vi "Find Lowest F-Cost.vi"(6 "Closed List In":T1(array[cluster]), 8 "error in (no error)":errorcluster, 10 "Open List":T1(array[cluster])) -> (0 "error out":errorcluster, 1 "Square with Parent":T2, 2 "Square":cluster{"X":dbl, "Y":dbl}, 3 "Open List Out":T1(array[cluster]), 4 "Closed List Out":T1(array[cluster]))   [LabVIEW 2009]
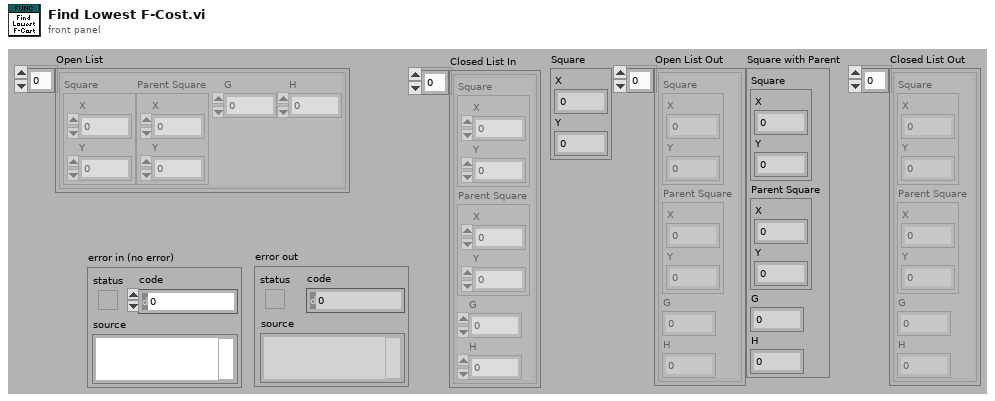
[diagram p1: front panel]
types:
  T1 = cluster{"Square":cluster{"X":dbl, "Y":dbl}, "Parent Square":cluster{"X":dbl, "Y":dbl}, "G":dbl, "H":dbl}[]
  T2 = cluster{"Square":cluster{"X":dbl, "Y":dbl}, "Parent Square":cluster{"X":dbl, "Y":dbl}, "G":dbl, "H":dbl}
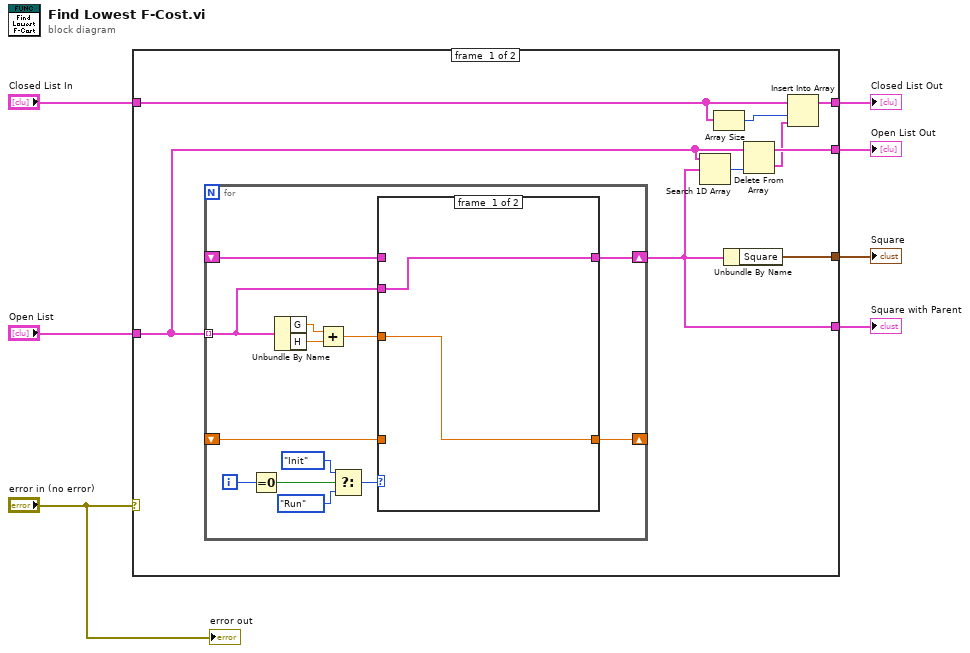
[diagram p0: block diagram]
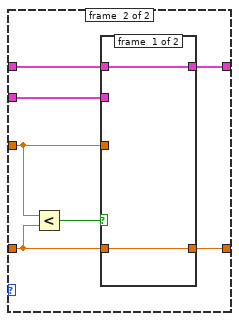
[diagram p2: hidden frame]
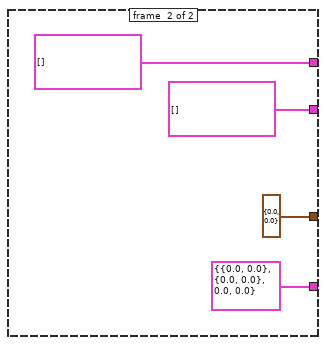
[diagram p4: hidden frame]
diagram:
  n1 = case shown="No Error" "error in (no error)" {
    tunnel: "Open List" -> [w16 _]
    tunnel: [w14 T1 [] ("Open List")] -> w5
    tunnel: [w13 cluster{"X":dbl, "Y":dbl} {"X"=0.0, "Y"=0.0} ("Square")] -> w4
    tunnel: [w12 T2 {"Square"={"X"=0.0, "Y"=0.0}, "Parent Square"={"X"=0.0, "Y"=0.0}, "G"=0.0, "H"=0.0} ("Cluster")] -> w3
    tunnel: "Closed List In" -> [w11 _]
    tunnel: [w8 T1 [] ("Closed List In")] -> w1
    frame #0 {
      n2 = for {
        tunnel: w16 -> [w19] mode=indexing
        shift-right: [w21] -> _
        shift-left: _ -> [w20]
        shift-right: [w18] -> w12
        shift-left: _ -> [w17]
        i -> [w24]
        n3 = Equal To 0?(x=w24) -> (x = 0?=w27:bool)
        n4 = Unbundle By Name(w19) -> ("G"=w29:dbl, "H"=w28:dbl)
        n5 = Add(x=w29, y=w28) -> (x+y=w22:dbl)
        n6 = Select(t=enum16{"Init", "Run"}."Init", s=w27, f=enum16{"Init", "Run"}."Run") -> (s? t:f=w23:enum16{"Init", "Run"})
        n7 = case shown="\"Run\"" w23 {
          tunnel: w22 -> [w31 w37]
          tunnel: [w31 w35] -> w21
          tunnel: w20 -> [_ w36]
          tunnel: w19 -> [w30 w32]
          tunnel: [w30 w34] -> w18
          tunnel: w17 -> [_ w33]
          frame #0 {
          }
          frame #1 {
            n8 = Less?(x=w37, y=w36) -> (x < y?=w38:bool)
            n9 = case shown="True" w38 {
              tunnel: w37 -> [_ w42]
              tunnel: w36 -> [w40 _]
              tunnel: [w40 w42] -> w35
              tunnel: [w39 w41] -> w34
              tunnel: w33 -> [w39 _]
              tunnel: w32 -> [_ w41]
              frame #0 {
              }
              frame #1 {
              }
            }
          }
        }
      }
      n10 = Search 1D Array(1D array=w16, element=w12) -> (index of element=w15:i32)  [unwired: 1 in]
      n11 = Array Size(array=w11) -> (size(s)=w10:i32)
      n12 = Unbundle By Name(w12) -> ("Square"=w13:cluster{"X":dbl, "Y":dbl})
      n13 = Delete From Array(array=w16, index=w15) -> (deleted portion=w9:T2, array with subset deleted=w14:T1)  [unwired: 1 in]
      n14 = Insert Into Array(array=w11, index=w10, new element=w9) -> (w8:T1)
    }
    frame #1 {
    }
  }
  "Square" <- w4
  "Open List Out" <- w5
  "Square with Parent" <- w3
  "Closed List Out" <- w1
  "error out" <- "error in (no error)"
